vi "RectToFRect-lv.vi"(1 "Rect":T2) -> (0 "FRect":T1)   [LabVIEW 2026, in "SDL3.lvlib" / "Rect.lvlib"]
doc: "<B>LV Implementation</B>\nSince the SDL function is inlined, we can't access in the shared library. So it's a LabVIEW implementation of the feature.\n\n<B>Summary</B>\nConvert an SDL_Rect to SDL_FRect"
uses:
  Rect.lvlib
  Rect--cluster.ctl
  FRect--cluster.ctl
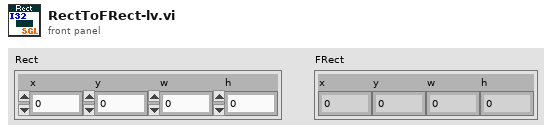
[diagram p1: front panel]
types:
  T1 = typedef "SDL3.lvlib/Rect.lvlib/FRect--cluster.ctl" = cluster{"x":sgl, "y":sgl, "w":sgl, "h":sgl}
  T2 = typedef "SDL3.lvlib/Rect.lvlib/Rect--cluster.ctl" = cluster{"x":i32, "y":i32, "w":i32, "h":i32}
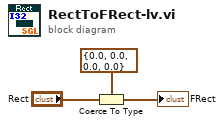
[diagram p0: block diagram]
diagram:
  n1 = Coerce To Type(0:"Rect", 1:T1 {"x"=0.0, "y"=0.0, "w"=0.0, "h"=0.0} ("FRect")) -> (2:→"FRect":T1)
